vi "Open.vi"(8 "error in (no error)":errorcluster, 11 "MelsecTCP in":refnum<class "InovanceSerialModbusRtu.lvclass">) -> (0 "error out":errorcluster, 3 "MelsecTCP out":refnum<class "InovanceSerialModbusRtu.lvclass">)   [LabVIEW 2020, in "HslCommunication.lvlib" / "InovanceSerialModbusRtu.lvclass"]
uses:
  InovanceSerialModbusRtu.lvclass
  InovanceSerialModbusRtu.lvclass/InovanceSerialModbusRtu.ctl
  E:/Git/Libraries/develop/HslCommunication/_Dependenciecs/HslCommunication.dll
  _Dependenciecs/HslCommunication.dll
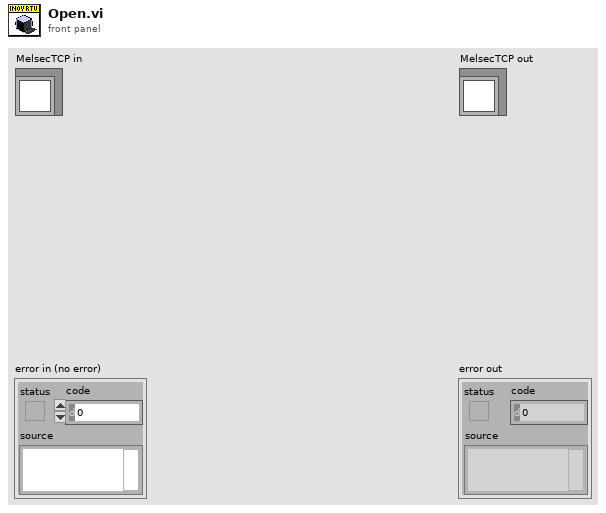
[diagram p1: front panel]
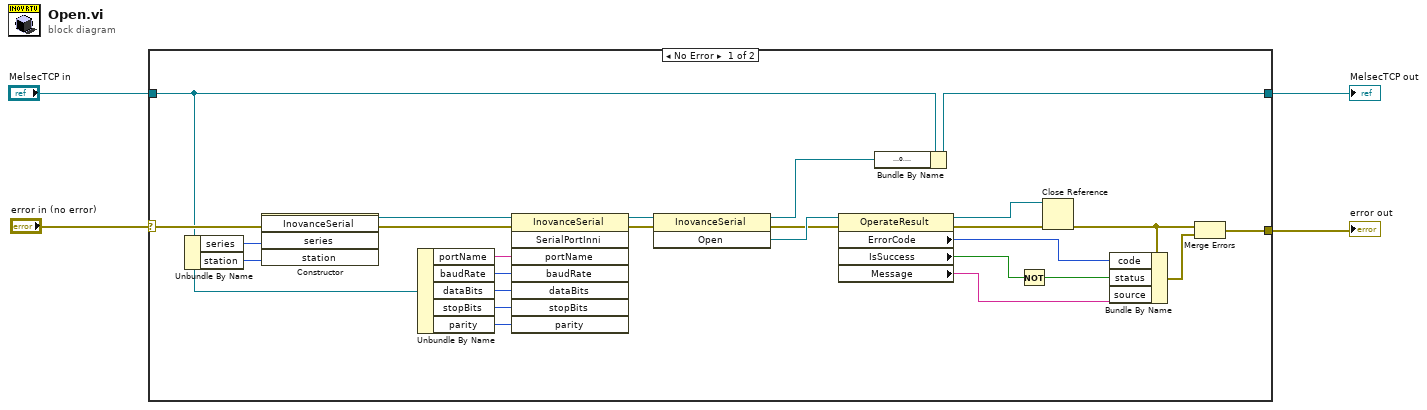
[diagram p0: block diagram]
diagram:
  n1 = case shown="No Error" "error in (no error)" {
    selector: "error in (no error)" -> [w17 w32]
    tunnel: "MelsecTCP in" -> [w11 w31]
    tunnel: [w30 w31] -> w1
    tunnel: [w24 w32] -> w2
    frame No Error {
      n2 = Unbundle By Name(w11) -> ("series"=w5:i32, "station"=w12:u8)
      n3 = constructor class="InovanceSerial"(error in=w17, "series"=w5, "station"=w12) -> (reference out=w21:refnum<k24>, error out=w20:errorcluster)  [unwired: 2 in, 3 out]
      n4 = Unbundle By Name(w11) -> ("portName"=w6:string, "baudRate"=w10:i32, "dataBits"=w9:i32, "stopBits"=w8:i32, "parity"=w7:i32)
      n5 = invoke class="InovanceSerial" method="SerialPortInni"(reference=w21, error in=w20, "portName"=w6, "baudRate"=w10, "dataBits"=w9, "stopBits"=w8, "parity"=w7) -> (reference out=w18:refnum<k24>, error out=w15:errorcluster)  [unwired: 1 in, 6 out]
      n6 = invoke class="InovanceSerial" method="Open"(reference=w18, error in=w15) -> (reference out=w16:refnum<k24>, error out=w13:errorcluster, "Open"=w14:refnum<k24>)  [unwired: 1 in]
      n7 = property class="OperateResult"(reference=w14, error in=w13) -> (reference out=w23:refnum<k24>, error out=w22:errorcluster, "ErrorCode"=w27:i32, "IsSuccess"=w19:bool, "Message"=w25:string)
      n8 = Bundle By Name(cluster=w11, "reference"=w16) -> (w30:refnum<class "InovanceSerialModbusRtu.lvclass">)
      n9 = Not(x=w19) -> (.not. x?=w26:bool)
      n10 = Close Reference(reference=w23, error in (no error)=w22) -> (error out=w28:errorcluster)
      n11 = Bundle By Name(cluster=w28, "code"=w27, "status"=w26, "source"=w25) -> (w29:errorcluster)
      n12 = Merge Errors(w28, w29) -> (w24:errorcluster)
    }
    frame Error {
    }
  }
  "error out" <- w2
  "MelsecTCP out" <- w1
